vi "Test - Class to Cluster Round Trip.vi"(8 "error in":errorcluster) -> (0 "error out":errorcluster)   [LabVIEW 2020, in "TEST - JKI JSON Object Serialization.lvlib"]
uses:
  TEST - JKI JSON Object Serialization.lvlib
  source/examples/Class1/Class1.lvclass
  <vilib>/addons/_JKI Toolkits/Caraya/classes/Test/Test.lvclass
  source/library/JKI JSON Object Serialization.lvlib
  <vilib>/addons/_JKI Toolkits/Caraya/classes/Assert/Assert.lvclass
panel:
  out "x = y?":bool
  out "JSON String":string
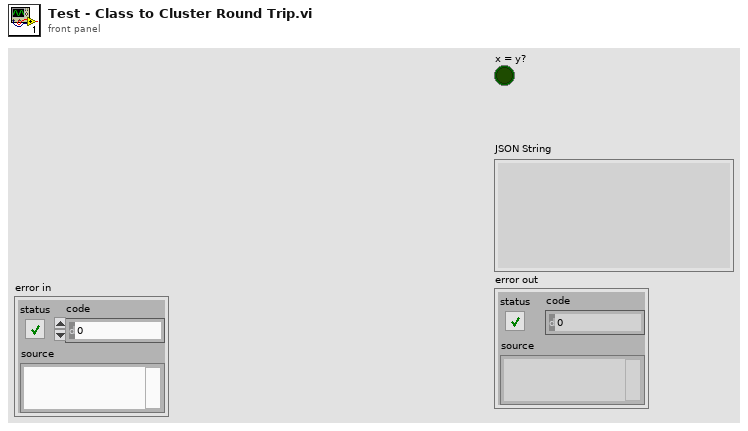
[diagram p1: front panel]
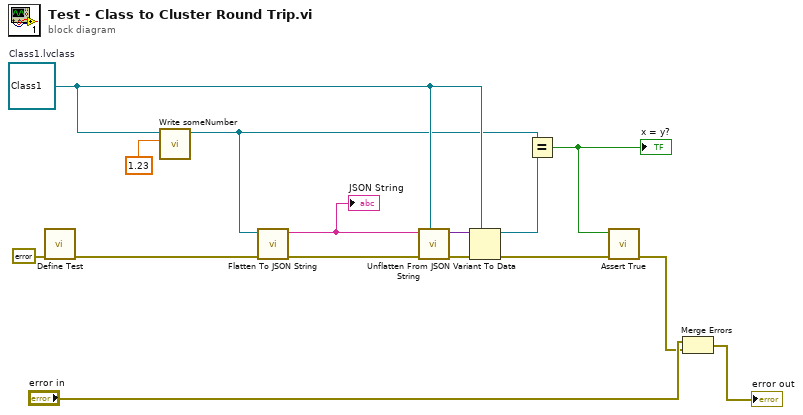
[diagram p0: block diagram]
diagram:
  w7 = refnum<class "Class1.lvclass"> refnum  # Class1.lvclass
  n1 = call <vilib>:"Define Test.vi"("error in (no error)"=errorcluster {"status"=FALSE, "code"=0, "source"=""}) -> ("error out"=w3:errorcluster)  [unwired: 9 in, 1 out]
  n2 = call-dynamic "Write someNumber.vi"("someNumber"=1.23, "Test1 in"=w7) -> ("Test1 out"=w5:refnum<class "Class1.lvclass">)  [unwired: 8 in, 1 out]
  n3 = call "Flatten To JSON String.vi"("error in (no error)"=w3, "Variant"=w5) -> ("error out"=w11:errorcluster, "JSON String"=w10:string)  [unwired: 8 in]
  "JSON String" <- w10
  n4 = call "Unflatten From JSON String.vi"("Type and Defaults"=w7, "error in (no error)"=w11, "JSON String"=w10) -> ("error out"=w9:errorcluster, "Variant"=w8:variant)  [unwired: 7 in]
  n5 = Variant To Data(error in=w9, type=w7, Variant=w8) -> (data=w6:refnum<class "Class1.lvclass">, error out=w4:errorcluster)
  n6 = Equal?(x=w5, y=w6) -> (x = y?=w1:bool)
  "x = y?" <- w1
  n7 = call <vilib>:"Assert True.vi"("error in (no error)"=w4, "True?"=w1) -> ("error out"=w2:errorcluster)  [unwired: 8 in, 1 out]
  n8 = Merge Errors("error in", w2) -> (→"error out":errorcluster)
